vi "Identity ID.vi"(11 "DataHandlerIdentity in":refnum<class "DataHandlerIdentity.lvclass">) -> (2 "ID":string)   [LabVIEW 2020, in "Volatus.lvlib" / "DataHandlerIdentity.lvclass"]
uses:
  DataHandlerIdentity.lvclass
  DataHandlerIdentity.lvclass/DataHandlerIdentity.ctl
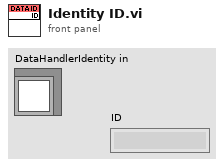
[diagram p1: front panel]
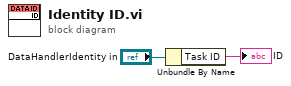
[diagram p0: block diagram]
diagram:
  n1 = Unbundle By Name("DataHandlerIdentity in") -> ("Task ID"=→"ID":string)
